vi "Get Value By Key.vi"(10 "Key":string, 11 "Key-Value Pairs":T1[](array[typedef])) -> (2 "Value":string)   [LabVIEW 2012]
uses:
  Key-Value Pair.ctl
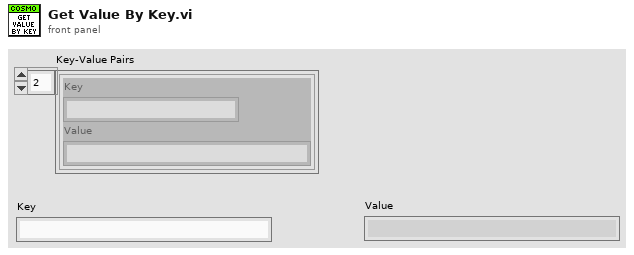
[diagram p1: front panel]
types:
  T1 = typedef "Key-Value Pair.ctl" = cluster{"Key":string, "Value":string}
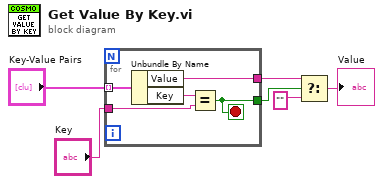
[diagram p0: block diagram]
diagram:
  n1 = for {
    tunnel: "Key-Value Pairs" -> [w11] mode=indexing
    tunnel: "Key" -> [w9]
    tunnel: [w8] -> w3
    tunnel: [w7] -> w4
    stop <- w7 stop-if-true
    n2 = Unbundle By Name(w11) -> ("Value"=w8:string, "Key"=w10:string)
    n3 = Equal?(x=w10, y=w9) -> (x = y?=w7:bool)
  }
  n4 = Select(t=w3, s=w4, f="") -> (s? t:f=→"Value":string)
